vi "SetParam.vi"(8 "error in (no error)":errorcluster caption="entrée d'erreur (pas d'erreur)", 10 "pairwise_distances_chunked":T1={"reduce_func"="None", "metric "="euclidean", "n_jobs"="None", "working_memory"="None"}, 11 "Pairwise_distances_chunked.lvclass":refnum<class "Pairwise_distances_chunked.lvclass">) -> (0 "error out":errorcluster caption="sortie d'erreur", 3 "Pairwise_distances_chunked.lvclass":refnum<class "Pairwise_distances_chunked.lvclass">)   [LabVIEW 2020, in "Pairwise_distances_chunked.lvclass"]
doc: "Set Parameters"
uses:
  Pairwise_distances_chunked.lvclass
  Pairwise_distances_chunked.lvclass/Pairwise_distances_chunked.ctl
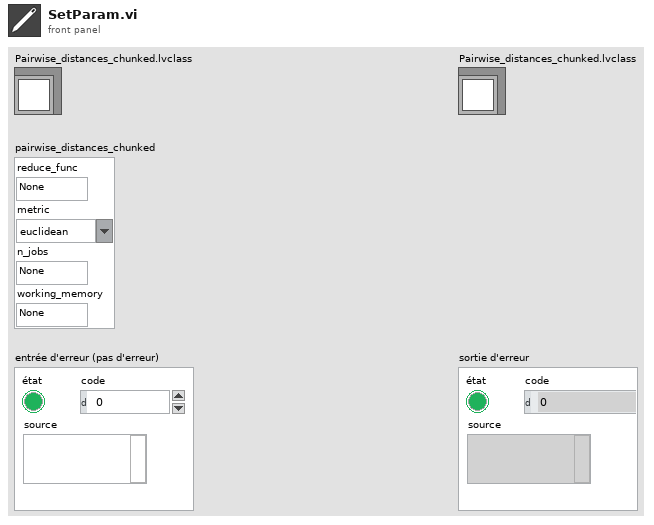
[diagram p1: front panel]
types:
  T1 = cluster{"reduce_func":string, "metric ":string, "n_jobs":string, "working_memory":string}
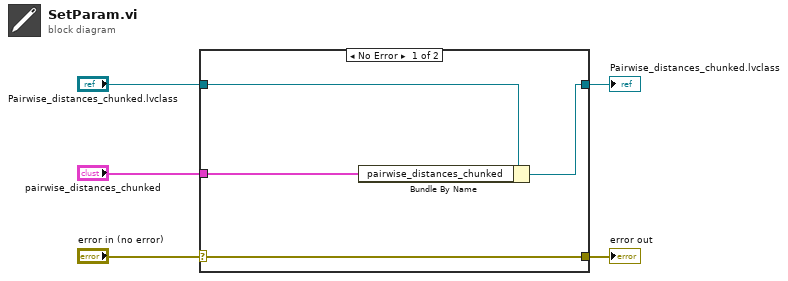
[diagram p0: block diagram]
diagram:
  n1 = case shown="No Error" "error in (no error)" {
    selector: "error in (no error)" -> [w9 w10]
    tunnel: [w9 w10] -> w4
    tunnel: [w7 w11] -> w2
    tunnel: "Pairwise_distances_chunked.lvclass" -> [w8 w11]
    tunnel: "pairwise_distances_chunked" -> [w6 _]
    frame No Error {
      n2 = Bundle By Name(cluster=w8, "pairwise_distances_chunked"=w6) -> (w7:refnum<class "Pairwise_distances_chunked.lvclass">)
    }
    frame Error {
    }
  }
  "error out" <- w4
  "Pairwise_distances_chunked.lvclass" <- w2
